vi "USRP Packet Transmitter_Queue.vi"() -> ()   [LabVIEW 2013]
uses:
  <vilib>/addons/Modulation/Digital/General/MT Generate PSK System Parameters(M).vi
  <vilib>/addons/Modulation/niDMT.lvlib
panel:
  out "error out":errorcluster
  out "Transmitted Signal":cluster{"t0":dbl, "dt":dbl, "Y":dbl[]}(graph)
  in  "Sample Rate [s/sec]":dbl=400000.0 format="%#.6p"
  in  "Modulation type":string(combo)="QPSK"
  in  "Pulse Shaping\nFilter Parameters":T1={"Alpha"=0.5, "Filter Length"=6, "TX Filter"=enum."Root Raised Cos"} caption="Pulse Shaping Filter" {"Alpha" format="%.2f"}
  out "Symbol Rate [symbols/sec]":dbl=50000.0 format="%#.6p"
  in  "Message Text":string="Two roads diverged in a yellow wood,\nAnd sorry I could not travel both\nAnd be one traveler, long I stood\nAnd looked down one as far as I could\nTo where it bent in the undergrowth.\n\nThen took the other, as just as fair,\nAnd having perhaps the better claim,\nBecause it was grassy and wanted wear;\nThough as for that the passing there\nHad worn them really about the same.\n\nAnd both that morning equally lay\nIn leaves no step had trodden black.\nOh, I kept the first for another day!\nYet knowing how way leads on to way,\nI doubted if I should ever come back.\n\nI shall be telling this with a sigh\nSomewhere ages and ages hence:\nTwo roads diverged in a wood, and I--\nI took the one less traveled by,\nAnd that has made all the difference.\n"
  out "Constellation Graph":cluster{dbl[], dbl[]}(graph)
  in  "Packet Parameters":T2={"Guard Bits "=30, "Sync Bits"=20, "Message Bits"=128}
  in  "Packet Pad [samples]":i32=200
  in  "16-PSK System Parameters":T3={"Samples per Symbol"=8, "symbol map"=[], "Differential PSK"=enum."disable", "PSK type"=0} {"PSK type" items=["normal", "shifted", "offset"]; "symbol map" format="%.3f"}
  in  "8-PSK System Parameters":T3={"Samples per Symbol"=8, "symbol map"=[], "Differential PSK"=enum."disable", "PSK type"=0} {"PSK type" items=["normal", "shifted", "offset"]; "symbol map" format="%.3f"}
  in  "QPSK System Parameters":T3={"Samples per Symbol"=8, "symbol map"=[], "Differential PSK"=enum."disable", "PSK type"=0} {"PSK type" items=["normal", "shifted", "offset"]; "symbol map" format="%.3f"}
  in  "BPSK System Parameters":T3={"Samples per Symbol"=8, "symbol map"=[], "Differential PSK"=enum."disable", "PSK type"=0} {"PSK type" items=["normal", "shifted", "offset"]; "symbol map" format="%.3f"}
  in  "Queue Length":i32=10
  out "Number of Packets in Message":i32=46
  in  "PN sequence order\n for Sync Bits":i32=31 caption="PN sequence order (9)"
  in  "Message Type":bool=TRUE
  # "Packet Transmitter"
  # "Pad\nData"
  # "Guard\nBand"
  # "Sync\nSeq"
  # "Packet\nNumber"
  # "Data"
  # "Cyclic Pad"
  # "Guard\nBand"
  # "Sync\nSeq"
  # "Packet\nNumber"
  # "Data"
  # "Custom Text"
  # "PN Sequence"
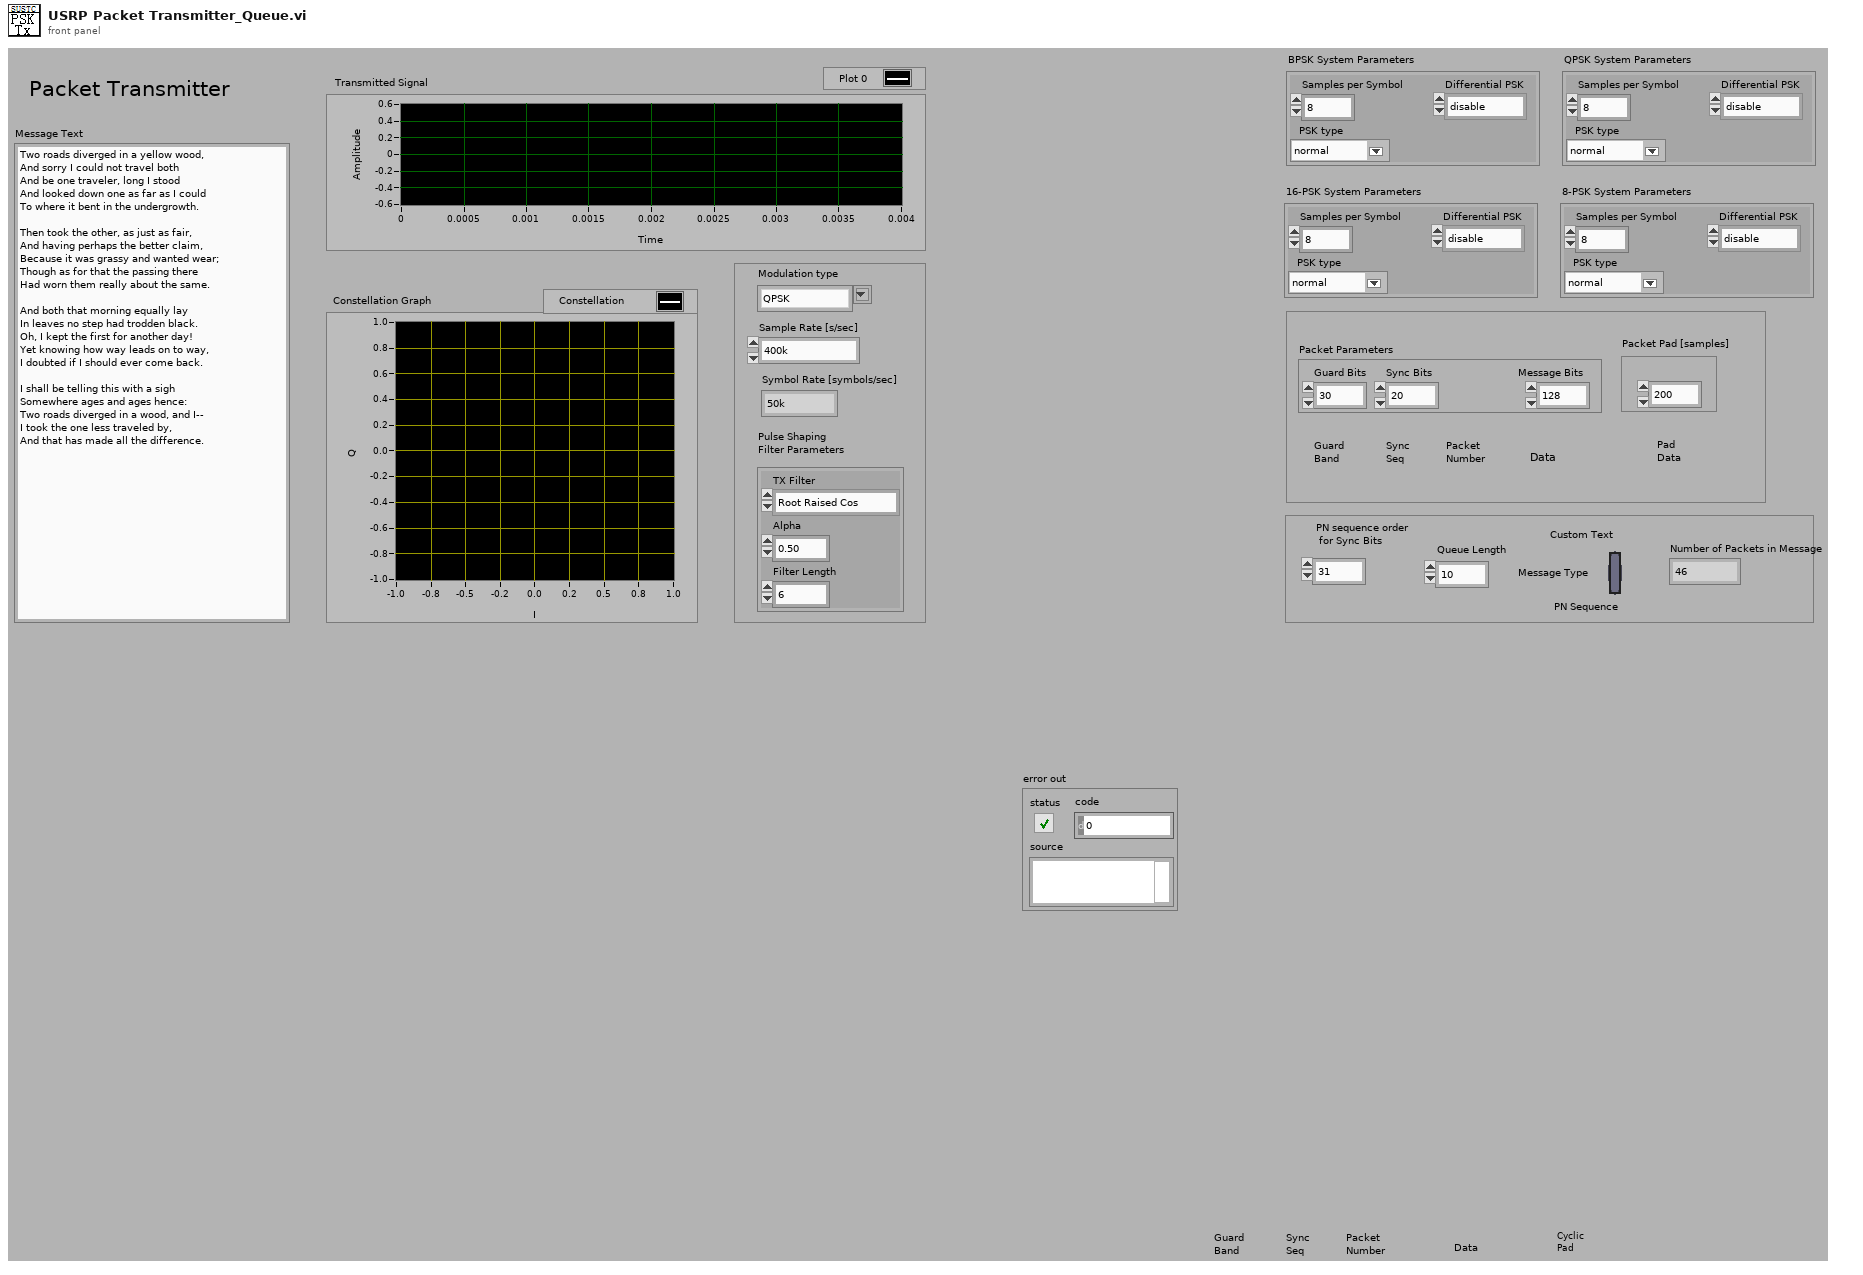
[diagram p1: front panel]
types:
  T1 = cluster{"Alpha":dbl, "Filter Length":i32, "TX Filter":enum16{"none", "Raised Cosine", "Root Raised Cos", "Gaussian"}}
  T2 = cluster{"Guard Bits ":i32, "Sync Bits":i32, "Message Bits":i32}
  T3 = cluster{"Samples per Symbol":i32, "symbol map":cdb[], "Differential PSK":enum16{"disable", "enable"}, "PSK type":u16}
  T4 = cluster{"samples per symbol (16)":i32, "symbol map":cdb[], "differential PSK":enum16{"disable", "enable"}, "PSK type":u16}
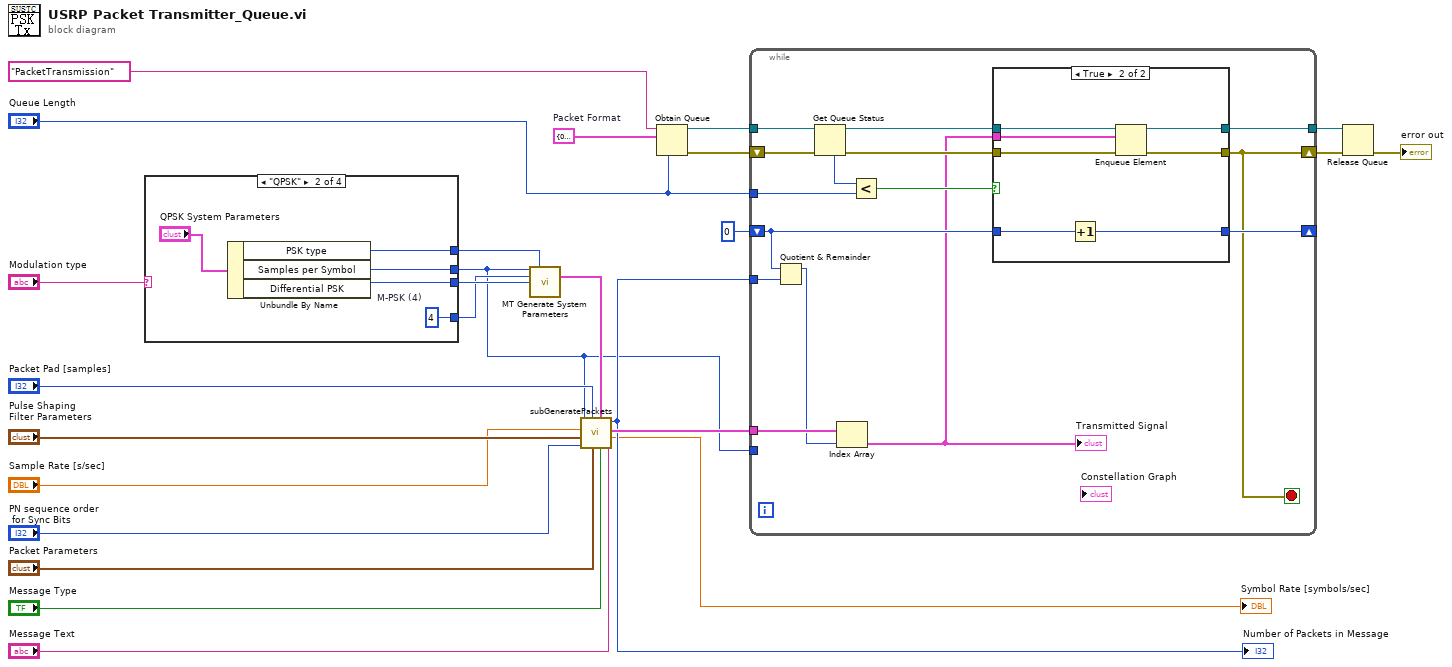
[diagram p0: block diagram]
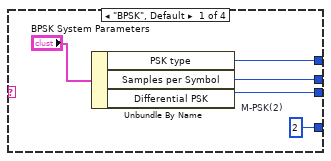
[diagram p3: hidden frame]
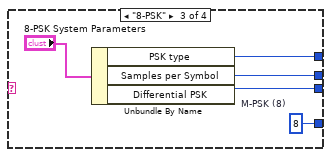
[diagram p4: hidden frame]
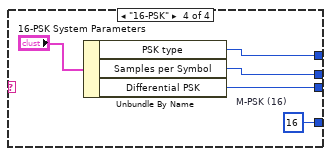
[diagram p5: hidden frame]
diagram:
  w4 = cluster{"t0":dbl, "dt":dbl, "Y":cdb[]} {"t0"=0.0, "dt"=0.0, "Y"=[]}  # Packet Format
  n1 = case shown="\"QPSK\"" "Modulation type" {
    tunnel: [w27 w31 w39 w45] -> w9
    tunnel: [w28 w33 w38 w44] -> w25
    tunnel: [w30 w35 w37 w43] -> w19
    tunnel: [w29 w34 w40 w42] -> w13
    frame "BPSK", Default {
      w30 = 2  # M-PSK(2)
      n2 = Unbundle By Name("BPSK System Parameters") -> ("PSK type"=w29:u16, "Samples per Symbol"=w27:i32, "Differential PSK"=w28:enum16{"disable", "enable"})
    }
    frame "QPSK" {
      w35 = 4  # M-PSK (4)
      n3 = Unbundle By Name("QPSK System Parameters") -> ("PSK type"=w34:u16, "Samples per Symbol"=w31:i32, "Differential PSK"=w33:enum16{"disable", "enable"})
    }
    frame "8-PSK" {
      w37 = 8  # M-PSK (8)
      n4 = Unbundle By Name("8-PSK System Parameters") -> ("PSK type"=w40:u16, "Samples per Symbol"=w39:i32, "Differential PSK"=w38:enum16{"disable", "enable"})
    }
    frame "16-PSK" {
      w43 = 16  # M-PSK (16)
      n5 = Unbundle By Name("16-PSK System Parameters") -> ("PSK type"=w42:u16, "Samples per Symbol"=w45:i32, "Differential PSK"=w44:enum16{"disable", "enable"})
    }
  }
  n6 = call-poly <vilib>:"MT Generate System Parameters.vi"("samples per symbol (16)"=w9, "PSK type"=w13, "M-PSK (4)"=w19, "differential PSK"=w25) -> ("PSK system parameters"=w14:T4)  [unwired: 9 in, 2 out]
  n7 = call "subGeneratePackets.vi"("Message Text"="Message Text", "Message Type"="Message Type", "PSK system parameters"=w14, "Packet Parameters"="Packet Parameters", "Packet Pad \n[samples]"="Packet Pad [samples]", "PN sequence order\nfor Sync Bits"="PN sequence order\n for Sync Bits", "Pulse Shaping Filter Parameters"="Pulse Shaping\nFilter Parameters", "Tx IQ Sampling\nRate [s/sec]"="Sample Rate [s/sec]", "Samples per Symbol"=w9) -> ("Symbol Rate"=→"Symbol Rate [symbols/sec]":dbl, "Packets"=w21:cluster{"t0":dbl, "dt":dbl, "Y":cdb[]}[], "Number of Packets"=w18:i32)
  "Number of Packets in Message" <- w18
  n8 = Obtain Queue(max queue size (-1, unlimited)="Queue Length", name (unnamed)="PacketTransmission", element data type=w4) -> (queue out=w24:refnum<queue>, error out=w15:errorcluster)  [unwired: 2 in, 1 out]
  n9 = while {
    tunnel: w24 -> [w60]
    shift-right: [w54] -> _
    shift-left: 0 -> [w50]
    tunnel: w21 -> [w51]
    tunnel: "Queue Length" -> [w53]
    tunnel: w18 -> [w52]
    shift-right: [w48] -> w2
    shift-left: w15 -> [w55]
    tunnel: w9 -> [_]
    tunnel: [w47] -> w3
    stop <- w48 stop-if-true
    n10 = Quotient & Remainder(x=w50, y=w52) -> (x-y*floor(x/y)=w49:i32)  [unwired: 1 out]
    n11 = Get Queue Status(queue=w60, error in (no error)=w55) -> (queue out=w59:refnum<queue>, error out=w56:errorcluster, # elements in queue=w58:i32)  [unwired: 1 in, 5 out]
    n12 = Index Array(array=w51, index=w49) -> (element=w46:cluster{"t0":dbl, "dt":dbl, "Y":cdb[]})
    "Transmitted Signal" <- w46
    n13 = Less?(x=w58, y=w53) -> (x < y?=w57:bool)
    n14 = case shown="True" w57 {
      tunnel: w56 -> [w62 w70]
      tunnel: w59 -> [w61 w69]
      tunnel: [w62 w68] -> w48
      tunnel: w46 -> [_ w67]
      tunnel: w50 -> [w63 w66]
      tunnel: [w63 w65] -> w54
      tunnel: [w61 w64] -> w47
      frame False {
      }
      frame True {
        n15 = Increment(x=w66) -> (x+1=w65:i32)
        n16 = Enqueue Element(queue=w69, element=w67, error in (no error)=w70) -> (queue out=w64:refnum<queue>, error out=w68:errorcluster)  [unwired: 1 in, 1 out]
      }
    }
  }
  n17 = Release Queue(queue=w3, error in (no error)=w2) -> (error out=→"error out":errorcluster)  [unwired: 1 in, 2 out]
